vi "TCP_WriteBool.vi"(9 "Value Input":string, 11 "Name Input":string) -> (1 "Boolean Value":variant, 3 "Is Boolean?":bool)   [LabVIEW 2019]
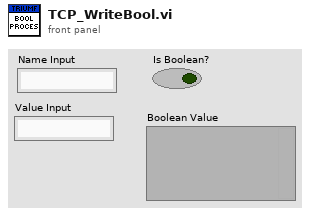
[diagram p1: front panel]
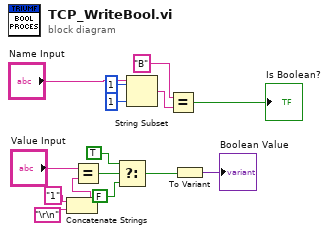
[diagram p0: block diagram]
diagram:
  n1 = Concatenate Strings("1" ("y"), "\r\n") -> (w1:string)
  n2 = Equal?(x="Value Input", y=w1) -> (x = y?=w8:bool)
  n3 = Select(t=TRUE ("x = y?"), s=w8, f=FALSE ("x = y?")) -> (s? t:f=w5:bool)
  n4 = String Subset(string="Name Input", offset (0)=1, length (rest)=1 ("length (rest)")) -> (substring=w12:string)
  n5 = Equal?(x="B", y=w12) -> (x = y?=→"Is Boolean?":bool)
  n6 = To Variant(anything=w5) -> (Variant=→"Boolean Value":variant)
